vi "Complementary Angle.vi"   [LabVIEW 2020, in "NI_AAL_Angle.lvlib"]
doc: "Calculates the complementary angle of the input angle.\n\nWire data to any of the angle inputs to determine the polymorphic instance to use or manually select the instance."
uses:
  <vilib>/Analysis/NI_AAL_Angle.lvlib
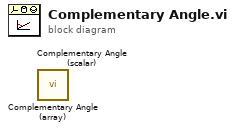
[diagram p0: block diagram]
diagram:
  n1 = call <vilib>:"Complementary Angle (array).vi"() -> ()  [unwired: 10 in, 2 out]
  n2 = call <vilib>:"Complementary Angle (scalar).vi"() -> ()  [unwired: 10 in, 2 out]
